vi "Configure Index of Refraction.vi"(8 "error in (no error)":errorcluster, 9 "Index of Refraction (0)":dbl, 10 "Channel (1: Channel 1)":i32(ring)=1 items=["Channel 1"=1, "Channel 1.1"=11, "Channel 1.2"=12, "Channel 1.3"=13, "Channel 1.4"=14, "Channel 2"=2, "Channel 2.1"=21, "Channel 2.2"=22, "Channel 2.3"=23, "Channel 2.4"=24, "Channel 3"=3, "Channel 3.1"=31, "Channel 3.2"=32, "Channel 3.3"=33, "Channel 3.4"=34, "Channel 4"=4, "Channel 4.1"=41, "Channel 4.2"=42, "Channel 4.3"=43, "Channel 4.4"=44], 11 "VISA resource name":refnum<visa-resource-name>) -> (0 "error out":errorcluster, 3 "VISA resource name out":refnum<visa-resource-name>)   [LabVIEW 2015, in "Micron Optics sm130.lvlib"]
doc: "Configures the optical index of refraction for the fiber on a specified channel, for use in the correction algorithm for the time-of-flight effects due to finite speed of light in optical fiber."
uses:
  Micron Optics sm130.lvlib
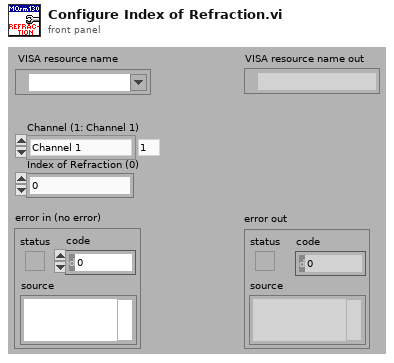
[diagram p1: front panel]
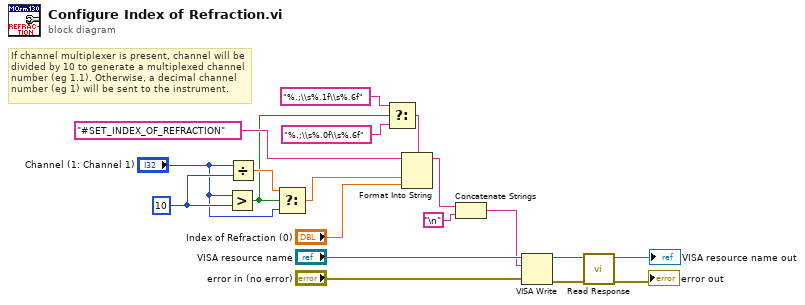
[diagram p0: block diagram]
diagram:
  w12 = 10 ("y")
  # "If channel multiplexer is present, channel will be divided by 10 to generate a multiplexed channel number (eg 1.1). Otherwise, a decimal channel number (eg 1) will be sent to the instrument."
  n1 = Greater?(x="Channel (1: Channel 1)", y=w12) -> (0:w6:bool)
  n2 = Divide(x="Channel (1: Channel 1)", y=w12) -> (x/y=w13:dbl)
  n3 = Select(t=w13, s=w6, f="Channel (1: Channel 1)") -> (s? t:f=w10:dbl)
  n4 = Select(t="%.;\\s%.1f\\s%.6f" ("format string"), s=w6, f="%.;\\s%.0f\\s%.6f" ("format string")) -> (s? t:f=w5:string)
  n5 = Format Into String(format string=w5, initial string="#SET_INDEX_OF_REFRACTION" ("input 1"), w10, "Index of Refraction (0)") -> (resulting string=w15:string)  [unwired: 1 in, 1 out]
  n6 = Concatenate Strings(w15, "\n") -> (w14:string)
  n7 = VISA Write(VISA resource name="VISA resource name", write buffer=w14, error in (no error)="error in (no error)") -> (VISA resource name out=w4:refnum<visa-resource-name>, error out=w3:errorcluster)  [unwired: 1 out]
  n8 = call "Read Response.vi"("error in (no error)"=w3, "VISA resource name"=w4) -> ("error out"=→"error out":errorcluster, "VISA resource name out"=→"VISA resource name out":refnum<visa-resource-name>)  [unwired: 7 in, 1 out]
